vi "Do.vi"(8 "error in (no error)":errorcluster, 10 "Actor in":refnum<class "Actor.lvclass">, 11 "ppanel_stream_TTTR Msg":refnum<class "ppanel_stream_TTTR Msg.lvclass">) -> (0 "error out":errorcluster, 2 "Actor out":refnum<class "Actor.lvclass">)   [LabVIEW 2015, in "ppanel_stream_TTTR Msg.lvclass"]
doc: "This VI delivers the message to the actor by calling the appropriate method(s) on the actor."
uses:
  ppanel_stream_TTTR Msg.lvclass
  <vilib>/ActorFramework/Actor/Actor.lvclass
  picoharp_panel/picoharp_panel.lvclass
  ppanel_stream_TTTR Msg.lvclass/ppanel_stream_TTTR Msg.ctl
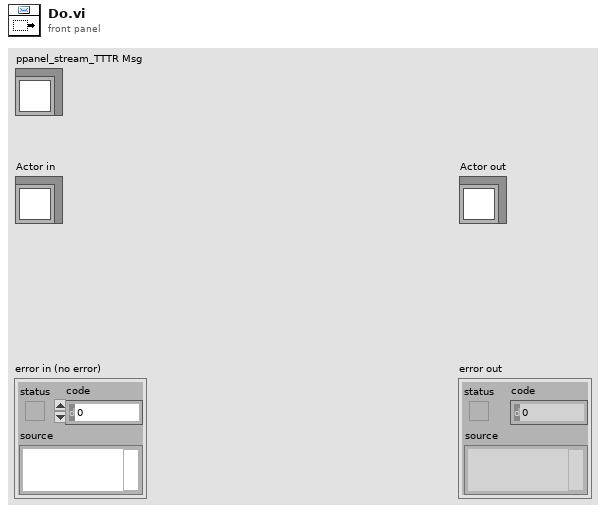
[diagram p1: front panel]
types:
  T1 = typedef "hydraharp_action_on_records.ctl" = enum16{"stream_to_file", "correlate", "stream to file and correlate"}
  T2 = typedef "record_type.ctl" = enum16{"Raw Stream", "Processed Records (hdf5)"}
  T3 = typedef "hpanel_correlation_settings.ctl" = cluster{"Lag Settings":T4, "Ch1":u8, "Ch2":u8}
  T4 = typedef "hydraharp_correlation_lag_settings.ctl" = cluster{"time_start":T5, "time_end":T5, "coarseness":i64}
  T5 = typedef "hydraharp_time_decades.ctl" = i64
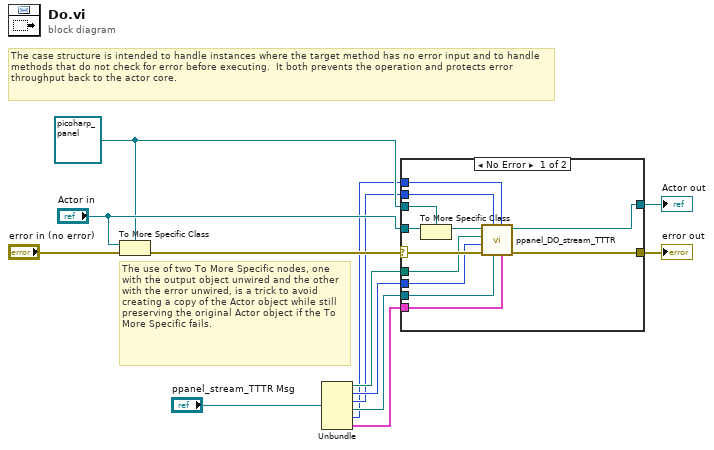
[diagram p0: block diagram]
diagram:
  w7 = refnum<class "picoharp_panel.lvclass"> refnum ("Actor in")
  # "The use of two To More Specific nodes, one with the output object unwired and the other with the error unwired, is a trick to avoid creating a copy of the Actor object while still preserving the original Actor object if the To More Specific fails."
  # "The case structure is intended to handle instances where the target method has no error input and to handle methods that do not check for error before executing.  It both prevents the operation and protects error throughput back to the actor core."
  n1 = To More Specific Class(target class=w7, reference="Actor in", error in="error in (no error)") -> (error out=w11:errorcluster)  [unwired: 1 out]
  n2 = Unbundle("ppanel_stream_TTTR Msg") -> (w6:path, w5:T1, w4:i32, w3:refnum<event-registration>, w2:T2, w1:T3)
  n3 = case shown="No Error" w11 {
    selector: w11 -> [w23 w27]
    tunnel: [w25 w27] -> w10
    tunnel: [w24 w26] -> w9
    tunnel: "Actor in" -> [w22 w26]
    tunnel: w7 -> [w21 _]
    tunnel: w6 -> [w19 _]
    tunnel: w5 -> [w18 _]
    tunnel: w4 -> [w17 _]
    tunnel: w3 -> [w16 _]
    tunnel: w2 -> [w15 _]
    tunnel: w1 -> [w14 _]
    frame No Error {
      n4 = To More Specific Class(target class=w21, reference=w22) -> (specific class reference=w20:refnum<class "picoharp_panel.lvclass">)  [unwired: 1 in, 1 out]
      n5 = call "ppanel_DO_stream_TTTR.vi"("Correlation_settings"=w14, "Record Type"=w15, "stop_fifo_event"=w16, "acq_time"=w17, "error in (no error)"=w23, "action_for_records"=w18, "fifo_stream_path"=w19, "hydraharp_panel in"=w20) -> ("error out"=w25:errorcluster, "hydraharp_panel out"=w24:refnum<class "picoharp_panel.lvclass">)  [unwired: 2 in]
    }
    frame Error {
      # "If type check fails, pass the original object out again."
    }
  }
  "error out" <- w10
  "Actor out" <- w9
